vi "Impedance_Single.vi"(0 "Measure Frequency":dbl=10000.0 format="%#.2p", 1 "Sampling Rate":dbl=250000.0 format="%#.3p", 11 "Number of runs":i32=5, 12 "Amplitude (pk)":dbl=0.05 format="%#.3p", 13 "Sampling Time":dbl=0.01 format="%#_6p") -> (4 "Impedance (Mag) - AvgInput":dbl=100001.51067957297 format="%#_3p", 6 "Impedance (Phase) - AvgInput":dbl=-0.6720456229115541 format="%#_3p", 8 "Inductance - AvgInput":dbl=-0.018667787926195056 format="%#_3p", 10 "Capacitance - AvgInput":dbl=1.3568986325926924e-08 format="%#_3p", 15 "Real (Z) - AvgInput":dbl=99994.6317029307 format="%#_3p")   [LabVIEW 2020]
uses:
  <vilib>/Analysis/baseanly.llb/Mean (CDB).vi
  <vilib>/Analysis/NI_AALBase.lvlib
panel:
  in  "TriggerLine":tag="/Dev3/ao/StartTrigger"
  in  "Current Ch":tag="Dev3/ai1"
  in  "Voltage Ch":tag="Dev3/ai0"
  in  "Output channels":tag="Dev3/ao0"
  out "St. Dev - R":dbl=19.698480410504242 format="%.2p"
  out "St. Dev - C":dbl=7.764141929346719e-10 format="%.2p"
  out "St. Dev - L":dbl=0.0010175327333416613 format="%.2p"
  in  "ESR":dbl=0.001
  in  "ESL":dbl=2.3e-07
  out "St. Dev - |Z|":dbl=19.72143726375669 format="%.4p"
  out "Current Run #":i32=99
  out "Time domain Signals":waveform(dbl)[](graph)=[{"t0"=timestamp(3724107274.8130174 s since 1904-01-01), "dt"=3.999999999999989e-06, "Y"=array[25000 elements], "attributes"=variant("NI_ChannelName"=variant(string "Dev3/ai0"), "NI_UnitDescription"=variant(string "Volts"))}, {"t0"=timestamp(3724107274.982843 s since 1904-01-01), "dt"=3.999999999999989e-06, "Y"=array[25000 elements], "attributes"=variant("NI_ChannelName"=variant(string "Dev3/ai1"), "NI_UnitDescription"=variant(string "Volts"))}]
  in  "UseCorrection":bool
  out "Real (Z)":dbl=99994.6034263936 format="%#_4p"
  out "Capacitance":dbl=1.3610699074622364e-08 format="%#_3p"
  out "Inductance":dbl=-0.01866779343788457 format="%#_3p"
  out "Impedance (Phase)":dbl=-0.672045691470684 format="%_3p"
  out "Impedance (Mag)":dbl=100001.50263935118 format="%_4p"
  in  "R_Shunt":dbl=10000.0
  out "Time domain Current\n(Measured Voltage)":waveform(dbl)(graph)={"t0"=timestamp(3724107274.982843 s since 1904-01-01), "dt"=3.999999999999989e-06, "Y"=array[25000 elements], "attributes"=variant("NI_ChannelName"=variant(string "Dev3/ai1"), "NI_UnitDescription"=variant(string "Volts"))}
  out "Time domain Voltage":waveform(dbl)(graph)={"t0"=timestamp(3724107274.8130174 s since 1904-01-01), "dt"=3.999999999999989e-06, "Y"=array[25000 elements], "attributes"=variant("NI_ChannelName"=variant(string "Dev3/ai0"), "NI_UnitDescription"=variant(string "Volts"))}
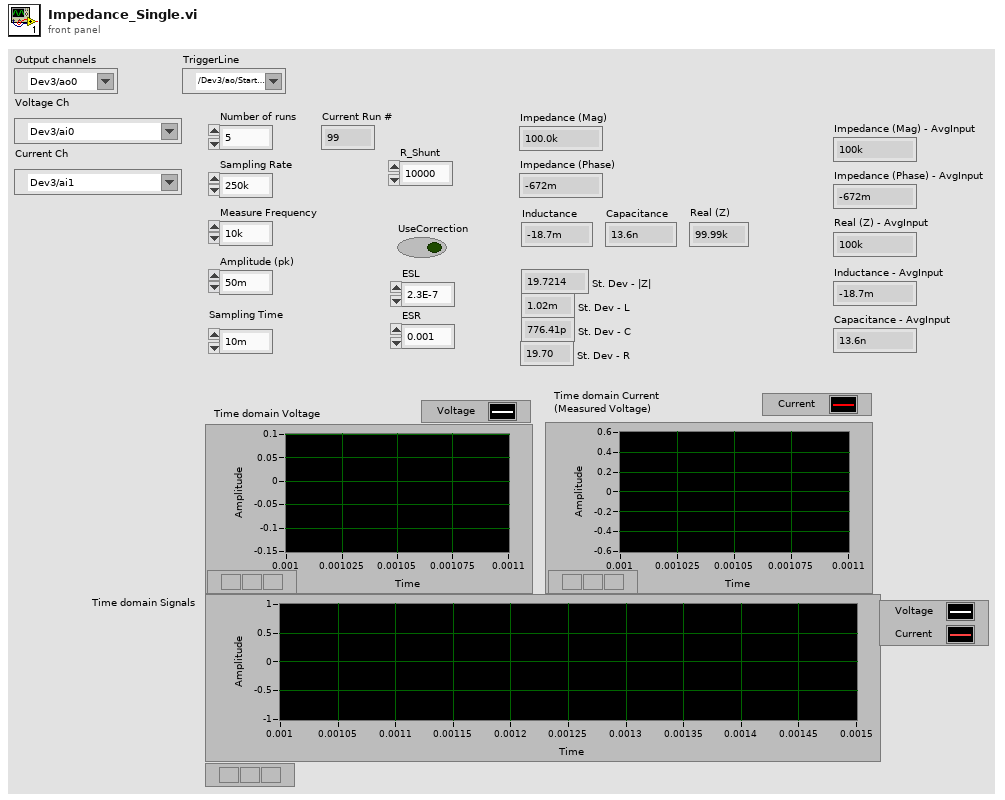
[diagram p1: front panel]
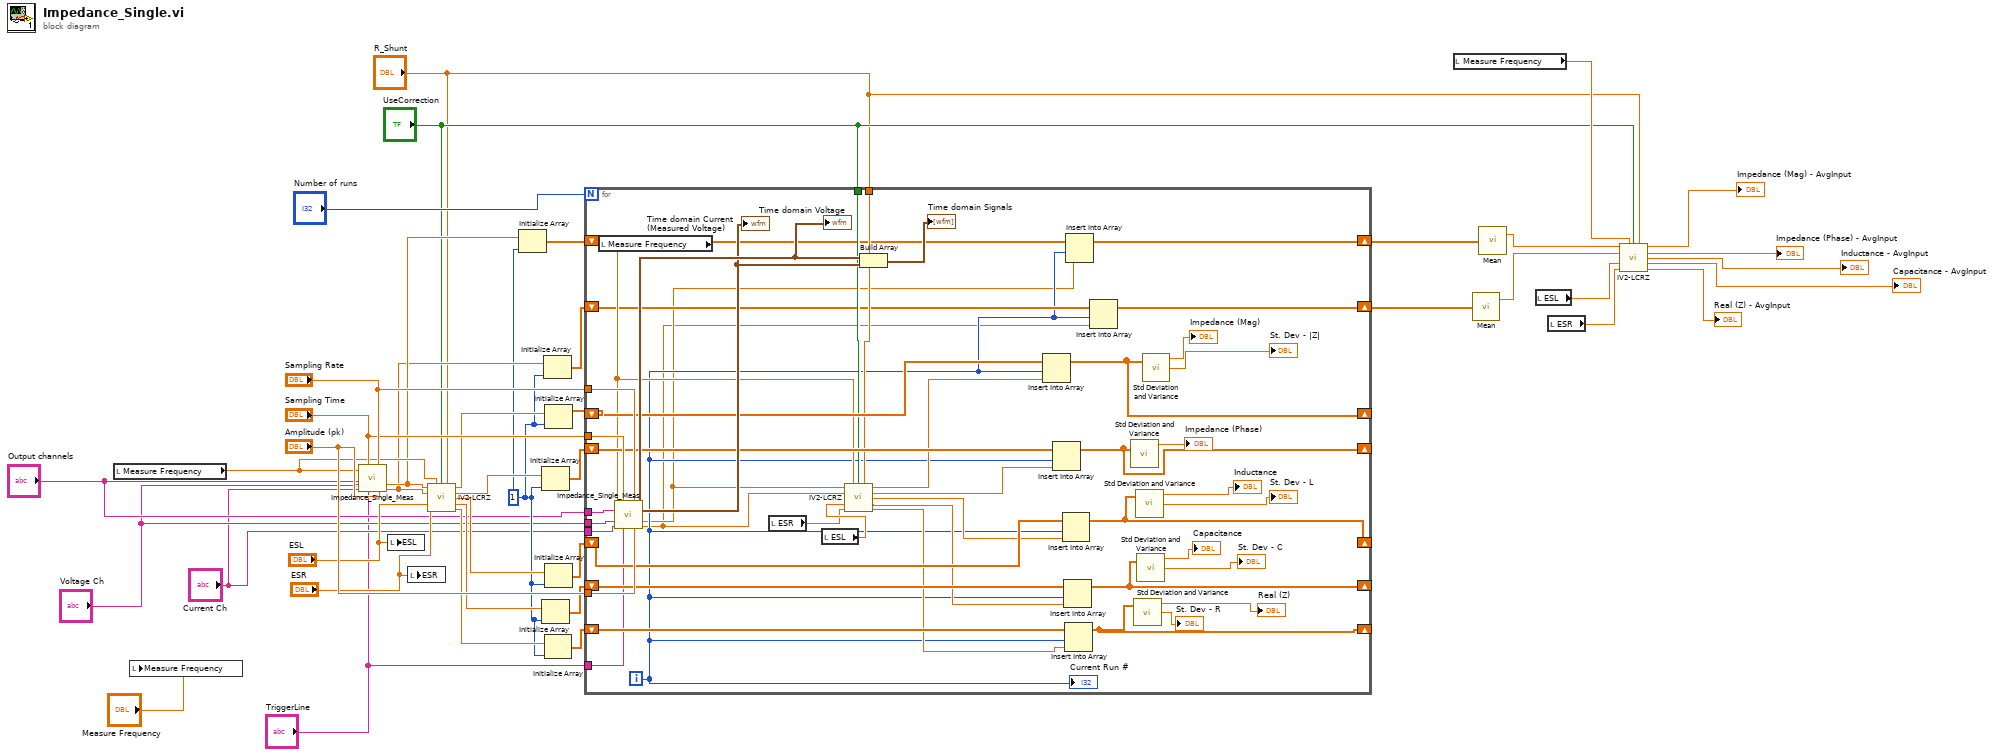
[diagram p0: block diagram]
diagram:
  w21 = 1 ("dimension size")
  n1 = local read "Measure Frequency"() -> (w32:dbl)
  n2 = local write "Measure Frequency"("Measure Frequency") -> ()
  n3 = call "Impedance_Single_Meas.vi"("frequency"=w32, "Time"="Sampling Time", "SampRate"="Sampling Rate", "Output channels"="Output channels", "Voltage Ch"="Voltage Ch", "Current Ch"="Current Ch", "TriggerLine"="TriggerLine", "amplitude"="Amplitude (pk)") -> ("Voltage Complex"=w23:cdb, "Current Complex"=w22:cdb)  [unwired: 4 in, 2 out]
  n4 = local write "ESL"("ESL") -> ()
  n5 = local write "ESR"("ESR") -> ()
  n6 = call "IV2-LCRZ.vi"("Voltage In"=w23, "Test Frequency"=w32, "UseCorrection"="UseCorrection", "R_Shunt"="R_Shunt", "Current In"=w22, "ESL"="ESL", "ESR"="ESR") -> ("Impedance (Mag)"=w31:dbl, "Impedance (Phase)"=w30:dbl, "Inductance"=w29:dbl, "Capacitance"=w28:dbl, "Real (Z)"=w27:dbl)  [unwired: 4 in]
  n7 = Initialize Array(w23, w21) -> (w20:cdb[])
  n8 = Initialize Array(w30, w21) -> (w35:dbl[])
  n9 = Initialize Array(w28, w21) -> (w25:dbl[])
  n10 = Initialize Array(w22, w21) -> (w19:cdb[])
  n11 = Initialize Array(w27, w21) -> (w24:dbl[])
  n12 = Initialize Array(w31, w21) -> (w36:dbl[])
  n13 = Initialize Array(w29, w21) -> (w26:dbl[])
  n14 = for {
    N: "Number of runs" -> [_]
    shift-right: [w56] -> _
    shift-left: w36 -> [w81]
    shift-right: [w55] -> _
    shift-left: w35 -> [w80]
    tunnel: "Sampling Rate" -> [w87]
    tunnel: "Sampling Time" -> [w86]
    tunnel: "Amplitude (pk)" -> [w85]
    shift-right: [w54] -> _
    shift-left: w26 -> [w79]
    shift-right: [w49] -> _
    shift-left: w25 -> [w78]
    shift-right: [w46] -> _
    shift-left: w24 -> [w77]
    tunnel: "UseCorrection" -> [w74]
    tunnel: "R_Shunt" -> [w73]
    shift-right: [w62] -> w18
    shift-left: w20 -> [w67]
    shift-right: [w61] -> w17
    shift-left: w19 -> [w66]
    tunnel: "Output channels" -> [w45]
    tunnel: "Voltage Ch" -> [w44]
    tunnel: "Current Ch" -> [w43]
    tunnel: "TriggerLine" -> [w42]
    i -> [w65]
    n15 = local read "Measure Frequency"() -> (w75:dbl)
    n16 = call "Impedance_Single_Meas.vi"("frequency"=w75, "Time"=w86, "SampRate"=w87, "Output channels"=w45, "Voltage Ch"=w44, "Current Ch"=w43, "TriggerLine"=w42, "amplitude"=w85) -> ("Time domain Voltage"=w83:waveform(dbl), "Time domain Current"=w82:waveform(dbl), "Voltage Complex"=w64:cdb, "Current Complex"=w63:cdb)  [unwired: 4 in]
    "Time domain Current\n(Measured Voltage)" <- w82
    "Time domain Voltage" <- w83
    n17 = local read "ESR"() -> (w60:dbl)
    n18 = local read "ESL"() -> (w76:dbl)
    n19 = call "IV2-LCRZ.vi"("Voltage In"=w64, "Test Frequency"=w75, "UseCorrection"=w74, "R_Shunt"=w73, "Current In"=w63, "ESL"=w76, "ESR"=w60) -> ("Impedance (Mag)"=w72:dbl, "Impedance (Phase)"=w71:dbl, "Inductance"=w70:dbl, "Capacitance"=w69:dbl, "Real (Z)"=w68:dbl)  [unwired: 4 in]
    n20 = Build Array(w83, w82) -> (→"Time domain Signals":waveform(dbl)[])
    n21 = Insert Into Array(array=w81, index=w65, new element=w72) -> (w56:dbl[])
    n22 = Insert Into Array(array=w80, index=w65, new element=w71) -> (w55:dbl[])
    n23 = Insert Into Array(array=w79, index=w65, new element=w70) -> (w54:dbl[])
    n24 = Insert Into Array(array=w78, index=w65, new element=w69) -> (w49:dbl[])
    n25 = Insert Into Array(array=w77, index=w65, new element=w68) -> (w46:dbl[])
    n26 = Insert Into Array(array=w67, index=w65, new element=w64) -> (w62:cdb[])
    n27 = Insert Into Array(array=w66, index=w65, new element=w63) -> (w61:cdb[])
    n28 = call <vilib>:"Std Deviation and Variance.vi"("X"=w55) -> ("mean"=→"Impedance (Phase)":dbl)  [unwired: 1 in, 2 out]
    n29 = call <vilib>:"Std Deviation and Variance.vi"("X"=w46) -> ("mean"=→"Real (Z)":dbl, "standard deviation"=→"St. Dev - R":dbl)  [unwired: 1 in, 1 out]
    n30 = call <vilib>:"Std Deviation and Variance.vi"("X"=w54) -> ("mean"=→"Inductance":dbl, "standard deviation"=→"St. Dev - L":dbl)  [unwired: 1 in, 1 out]
    n31 = call <vilib>:"Std Deviation and Variance.vi"("X"=w49) -> ("mean"=→"Capacitance":dbl, "standard deviation"=→"St. Dev - C":dbl)  [unwired: 1 in, 1 out]
    n32 = call <vilib>:"Std Deviation and Variance.vi"("X"=w56) -> ("mean"=→"Impedance (Mag)":dbl, "standard deviation"=→"St. Dev - |Z|":dbl)  [unwired: 1 in, 1 out]
    "Current Run #" <- w65
  }
  n33 = local read "Measure Frequency"() -> (w12:dbl)
  n34 = call-poly <vilib>:"Mean.vi"("X"=w17) -> ("mean"=w15:cdb)  [unwired: 1 out]
  n35 = call-poly <vilib>:"Mean.vi"("X"=w18) -> ("mean"=w16:cdb)  [unwired: 1 out]
  n36 = local read "ESL"() -> (w14:dbl)
  n37 = local read "ESR"() -> (w13:dbl)
  n38 = call "IV2-LCRZ.vi"("Voltage In"=w16, "Test Frequency"=w12, "UseCorrection"="UseCorrection", "R_Shunt"="R_Shunt", "Current In"=w15, "ESL"=w14, "ESR"=w13) -> ("Impedance (Mag)"=→"Impedance (Mag) - AvgInput":dbl, "Impedance (Phase)"=→"Impedance (Phase) - AvgInput":dbl, "Inductance"=→"Inductance - AvgInput":dbl, "Capacitance"=→"Capacitance - AvgInput":dbl, "Real (Z)"=→"Real (Z) - AvgInput":dbl)  [unwired: 4 in]
